vi "Test Basic Operations.vi"() -> ()   [LabVIEW 2014]
uses:
  <vilib>/Aledyne-TSXperts/Arduino Compatible Compiler for LabVIEW/Arduino Compatible Compiler for LabVIEW.lvlib
  <vilib>/Aledyne-TSXperts/Arduino Compatible Compiler for LabVIEW/addons/Complex Numbers/Complex Numbers.lvlib
panel:
  out "error out":errorcluster
  in  "error in (no error)":errorcluster
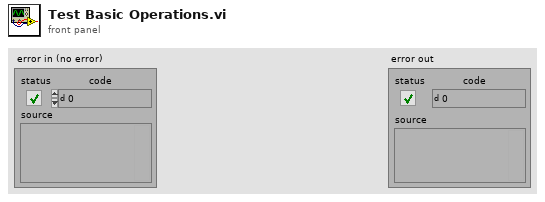
[diagram p1: front panel]
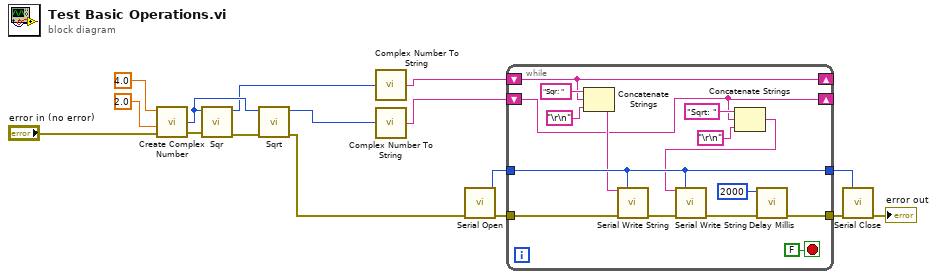
[diagram p0: block diagram]
diagram:
  n1 = call <vilib>:"Create Complex Number.vi"("Error In"="error in (no error)", "Imag"=2.0, "Real"=4.0) -> ("Error Out"=w8:errorcluster, "Complex"=w6:u32)  [unwired: 2 in]
  n2 = call <vilib>:"Sqr.vi"("Error In"=w8, "A"=w6) -> ("Error Out"=w7:errorcluster, "sqr(A)"=w3:u32)  [unwired: 8 in]
  n3 = call <vilib>:"Sqrt.vi"("Error In"=w7, "A"=w6) -> ("Error Out"=w4:errorcluster, "sqrt(A)"=w5:u32)  [unwired: 8 in]
  n4 = call <vilib>:"Complex Number To String.vi"("Complex number"=w3) -> ("String complex num."=w1:string)
  n5 = call <vilib>:"Complex Number To String.vi"("Complex number"=w5) -> ("String complex num."=w2:string)
  n6 = call <vilib>:"Serial Open.vi"("error in (no error)"=w4) -> ("Instance"=w14:u8, "error out"=w16:errorcluster)  [unwired: 13 in]
  n7 = while {
    tunnel: w16 -> [w27]
    tunnel: [w29] -> w15
    tunnel: w14 -> [w25]
    tunnel: [w25] -> w13
    shift-right: [w19] -> _
    shift-left: w1 -> [w19]
    shift-right: [w17] -> _
    shift-left: w2 -> [w17]
    stop <- FALSE stop-if-true
    n8 = Concatenate Strings("Sqr: " ("string"), w19, "\r\n") -> (w22:string)
    n9 = call <vilib>:"Serial Write String.vi"("String"=w22, "Instance"=w25, "error in (no error)"=w27) -> ("error out"=w26:errorcluster)  [unwired: 12 in]
    n10 = Concatenate Strings("Sqrt: " ("string"), w17, "\r\n") -> (w21:string)
    n11 = call <vilib>:"Serial Write String.vi"("String"=w21, "Instance"=w25, "error in (no error)"=w26) -> ("error out"=w30:errorcluster)  [unwired: 12 in]
    n12 = call <vilib>:"Delay Millis.vi"("error in (no error)"=w30, "delay"=u32 2000) -> ("error out"=w29:errorcluster)  [unwired: 9 in]
  }
  n13 = call <vilib>:"Serial Close.vi"("Instance"=w13, "error in (no error)"=w15) -> ("error out"=→"error out":errorcluster)  [unwired: 13 in]
